vi "MTS_CalcMeasTime.vi"(0 "Image Measurent Parameters":T1, 1 "ht3 header in":T2={"Comment"="", "Binning"=0, "Offset"=0, "AcquisitionTime (ms)"=0, "HardwareSerial"=0, "SyncDivider"=0, "Resolution (ps)"=0.0, "InpRate0"=0, "InpRate1"=0, "CFD Settings"={"Sync Level"=150, "Sync ZeroX"=10, "Sync Offset"=-1000, "Chan Settings"=[{"CHx Level"=50, "CHx ZeroX"=10, "CHx Offset"=0}, {"CHx Level"=50, "CHx ZeroX"=10, "CHx Offset"=0}, {"CHx Level"=50, "CHx ZeroX"=10, "CHx Offset"=0}, {"CHx Level"=50, "CHx ZeroX"=10, "CHx Offset"=0}]}, "ModuleInfo"=[], "BaseResolution (ps)"=0.0, "RefClockSource"=0, "ChanInfo"=[], "SyncRate"=0, "InputsEnabled"=0}, 7 "Measurement time [s]":i32, 11 "Count Rate":i32) -> (3 "ht3 header out":T2={"Comment"="", "Binning"=0, "Offset"=0, "AcquisitionTime (ms)"=0, "HardwareSerial"=0, "SyncDivider"=0, "Resolution (ps)"=0.0, "InpRate0"=0, "InpRate1"=0, "CFD Settings"={"Sync Level"=150, "Sync ZeroX"=10, "Sync Offset"=-1000, "Chan Settings"=[{"CHx Level"=50, "CHx ZeroX"=10, "CHx Offset"=0}, {"CHx Level"=50, "CHx ZeroX"=10, "CHx Offset"=0}, {"CHx Level"=50, "CHx ZeroX"=10, "CHx Offset"=0}, {"CHx Level"=50, "CHx ZeroX"=10, "CHx Offset"=0}]}, "ModuleInfo"=[], "BaseResolution (ps)"=0.0, "RefClockSource"=0, "ChanInfo"=[], "SyncRate"=0, "InputsEnabled"=0}, 4 "Corrected Measurement time [s]":i32, 6 "Calc Acq. Time (ms)":i32, 10 "Overflow Interv. Time (s)":dbl, 15 "Pixel Time (Laser Pulses)":i32)   [LabVIEW 2011]
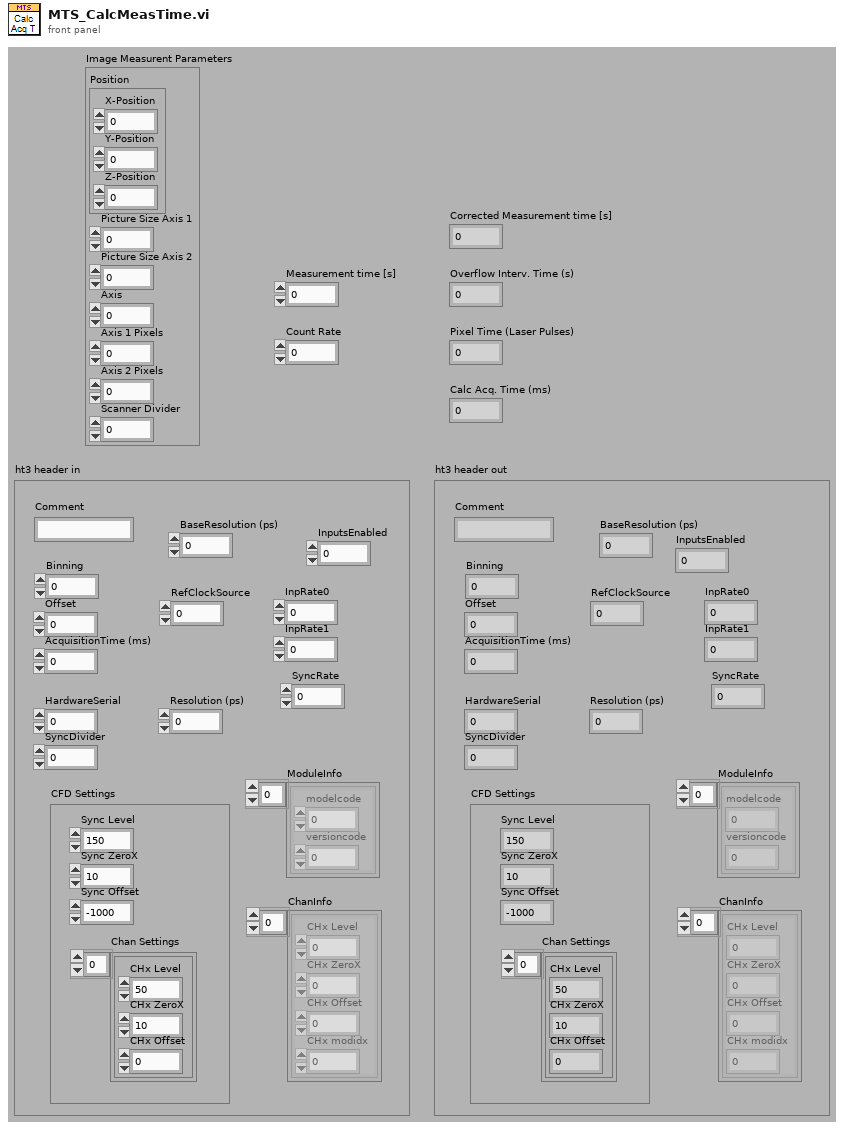
[diagram p1: front panel]
types:
  T1 = cluster{"Position":cluster{"X-Position":dbl, "Y-Position":dbl, "Z-Position":dbl}, "Picture Size Axis 1":dbl, "Picture Size Axis 2":dbl, "Axis":i32, "Axis 1 Pixels":u16, "Axis 2 Pixels":u16, "Scanner Divider":i32}
  T2 = cluster{"Comment":string, "Binning":i32, "Offset":i32, "AcquisitionTime (ms)":i32, "HardwareSerial":i32, "SyncDivider":i32, "Resolution (ps)":dbl, "InpRate0":i32, "InpRate1":i32, "CFD Settings":cluster{"Sync Level":i32, "Sync ZeroX":i32, "Sync Offset":i32, "Chan Settings":cluster{"CHx Level":i32, "CHx ZeroX":i32, "CHx Offset":i32}[]}, "ModuleInfo":cluster{"modelcode":i32, "versioncode":i32}[], "BaseResolution (ps)":dbl, "RefClockSource":i32, "ChanInfo":cluster{"CHx Level":i32, "CHx ZeroX":i32, "CHx Offset":i32, "CHx modidx":i32}[], "SyncRate":i32, "InputsEnabled":i64}
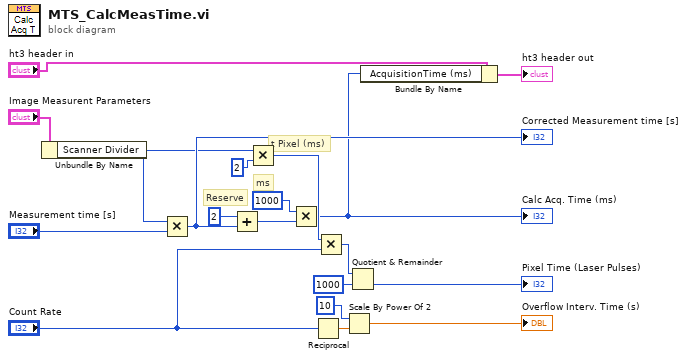
[diagram p0: block diagram]
diagram:
  # "t Pixel (ms)"
  # "ms"
  # "Reserve"
  n1 = Unbundle By Name("Image Measurent Parameters") -> ("Scanner Divider"=w1:i32)
  n2 = Multiply(x=w1, y="Measurement time [s]") -> (x*y=w7:i32)
  "Corrected Measurement time [s]" <- w7
  n3 = Add(x=2, y=w7) -> (x+y=w9:i32)
  n4 = Multiply(x=w1, y=2 ("x")) -> (x*y=w15:i32)
  n5 = Multiply(x=1000, y=w9) -> (x*y=w6:i32)
  "Calc Acq. Time (ms)" <- w6
  n6 = Reciprocal(x="Count Rate") -> (1/x=w13:dbl)
  n7 = Multiply(x=w15, y="Count Rate") -> (x*y=w17:i32)
  n8 = Scale By Power Of 2(n=10, x=w13) -> (x*2^n=→"Overflow Interv. Time (s)":dbl)
  n9 = Quotient & Remainder(x=w17, y=1000) -> (floor(x/y)=→"Pixel Time (Laser Pulses)":i32)  [unwired: 1 out]
  n10 = Bundle By Name(cluster="ht3 header in", "AcquisitionTime (ms)"=w6) -> (→"ht3 header out":T2)
